vi "test_libssh2_sftp_unlink_ex.vi"() -> ()   [LabVIEW 2017, in "integration_tests.lvlib"]
uses:
  integration_tests.lvlib
  support/support.lvlib
  libssh2/libssh2.lvlib
  <vilib>/PNR/Transparent Assertions/Transparent Assertions/Transparent Assertions.lvlib
panel:
  out "error out":errorcluster
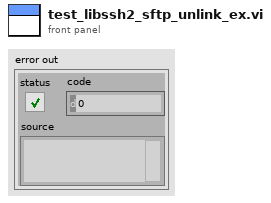
[diagram p1: front panel]
types:
  T1 = typedef "libssh2.lvlib/Session Refnum.ctl" = refnum<k1>
  T2 = typedef "libssh2.lvlib/SFTP Refnum.ctl" = refnum<k1>
  T3 = typedef "libssh2.lvlib/SFTP Handle Refnum.ctl" = refnum<k1>
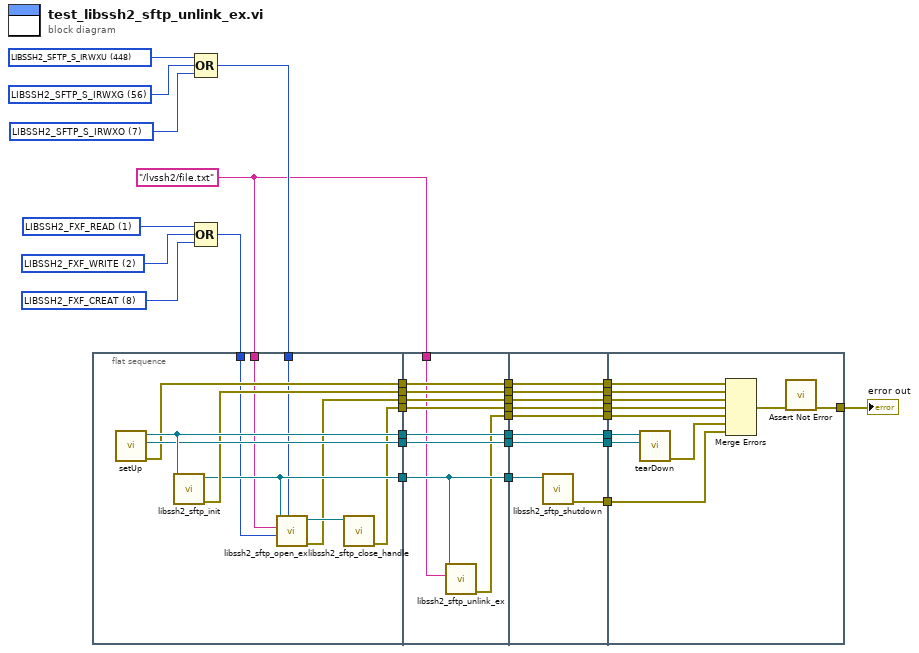
[diagram p0: block diagram]
diagram:
  w27 = u32 2 items=["LIBSSH2_FXF_READ"=1, "LIBSSH2_FXF_WRITE"=2, "LIBSSH2_FXF_APPEND"=4, "LIBSSH2_FXF_CREAT"=8, "LIBSSH2_FXF_TRUNC"=16, "LIBSSH2_FXF_EXCL"=32] ("flags")
  w28 = u32 1 items=["LIBSSH2_FXF_READ"=1, "LIBSSH2_FXF_WRITE"=2, "LIBSSH2_FXF_APPEND"=4, "LIBSSH2_FXF_CREAT"=8, "LIBSSH2_FXF_TRUNC"=16, "LIBSSH2_FXF_EXCL"=32] ("flags")
  w26 = u32 8 items=["LIBSSH2_FXF_READ"=1, "LIBSSH2_FXF_WRITE"=2, "LIBSSH2_FXF_APPEND"=4, "LIBSSH2_FXF_CREAT"=8, "LIBSSH2_FXF_TRUNC"=16, "LIBSSH2_FXF_EXCL"=32] ("flags")
  w3 = "/lvssh2/file.txt" ("filename")
  w30 = 7 items=["LIBSSH2_SFTP_S_IRWXU"=448, "LIBSSH2_SFTP_S_IRUSR"=256, "LIBSSH2_SFTP_S_IWUSR"=128, "LIBSSH2_SFTP_S_IXUSR"=64, "LIBSSH2_SFTP_S_IRWXG"=56, "LIBSSH2_SFTP_S_IRGRP"=32, "LIBSSH2_SFTP_S_IWGRP"=16, "LIBSSH2_SFTP_S_IXGRP"=8, "LIBSSH2_SFTP_S_IRWXO"=7, "LIBSSH2_SFTP_S_IROTH"=4, "LIBSSH2_SFTP_S_IWOTH"=2, "LIBSSH2_SFTP_S_IXOTH"=1] ("mode")
  w31 = 56 items=["LIBSSH2_SFTP_S_IRWXU"=448, "LIBSSH2_SFTP_S_IRUSR"=256, "LIBSSH2_SFTP_S_IWUSR"=128, "LIBSSH2_SFTP_S_IXUSR"=64, "LIBSSH2_SFTP_S_IRWXG"=56, "LIBSSH2_SFTP_S_IRGRP"=32, "LIBSSH2_SFTP_S_IWGRP"=16, "LIBSSH2_SFTP_S_IXGRP"=8, "LIBSSH2_SFTP_S_IRWXO"=7, "LIBSSH2_SFTP_S_IROTH"=4, "LIBSSH2_SFTP_S_IWOTH"=2, "LIBSSH2_SFTP_S_IXOTH"=1] ("mode")
  w32 = 448 items=["LIBSSH2_SFTP_S_IRWXU"=448, "LIBSSH2_SFTP_S_IRUSR"=256, "LIBSSH2_SFTP_S_IWUSR"=128, "LIBSSH2_SFTP_S_IXUSR"=64, "LIBSSH2_SFTP_S_IRWXG"=56, "LIBSSH2_SFTP_S_IRGRP"=32, "LIBSSH2_SFTP_S_IWGRP"=16, "LIBSSH2_SFTP_S_IXGRP"=8, "LIBSSH2_SFTP_S_IRWXO"=7, "LIBSSH2_SFTP_S_IROTH"=4, "LIBSSH2_SFTP_S_IWOTH"=2, "LIBSSH2_SFTP_S_IXOTH"=1] ("mode")
  n1 = flat-sequence {
    tunnel: [w44] -> w14
    tunnel: [w43] -> w13
    tunnel: [w40] -> w12
    tunnel: [w42] -> w11
    tunnel: [w41] -> w10
    tunnel: w29 -> [w39]
    tunnel: w3 -> [w38]
    tunnel: w25 -> [w37]
    tunnel: [w35] -> w9
    tunnel: [w34] -> w4
    tunnel: [w53] -> w19
    tunnel: [w52] -> w18
    tunnel: [w51] -> w17
    tunnel: [w50] -> w16
    tunnel: [w49] -> w15
    tunnel: [w48] -> w8
    tunnel: [w47] -> w5
    tunnel: w3 -> [w46]
    tunnel: w4 -> [w47]
    tunnel: w9 -> [w48]
    tunnel: w10 -> [w49]
    tunnel: w11 -> [w50]
    tunnel: w12 -> [w51]
    tunnel: w13 -> [w52]
    tunnel: w14 -> [w53]
    tunnel: [w45] -> w2
    tunnel: w19 -> [w62]
    tunnel: [w62] -> w24
    tunnel: w18 -> [w61]
    tunnel: [w61] -> w23
    tunnel: w17 -> [w58]
    tunnel: w16 -> [w60]
    tunnel: [w60] -> w22
    tunnel: w15 -> [w59]
    tunnel: [w59] -> w21
    tunnel: [w57] -> w20
    tunnel: w8 -> [w56]
    tunnel: [w56] -> w7
    tunnel: [w55] -> w6
    tunnel: w5 -> [w55]
    tunnel: w2 -> [w54]
    tunnel: [w54] -> w1
    tunnel: w24 -> [w73]
    tunnel: w23 -> [w72]
    tunnel: w22 -> [w71]
    tunnel: [w68] -> w33
    tunnel: w21 -> [w67]
    tunnel: w20 -> [w66]
    tunnel: w7 -> [w65]
    tunnel: w6 -> [w64]
    tunnel: w1 -> [w63]
    frame #0 {
      n2 = call "setUp.vi"() -> ("error out"=w42:errorcluster, "connection ID"=w43:refnum<k5>, "session"=w44:T1)  [unwired: 9 in]
      n3 = call "libssh2_sftp_init.vi"("session"=w44) -> ("error out"=w41:errorcluster, "sftp"=w40:T2)  [unwired: 9 in]
      n4 = call "libssh2_sftp_open_ex.vi"("mode"=w39, "flags"=w37, "filename"=w38, "sftp"=w40) -> ("error out"=w35:errorcluster, "sftp handle"=w36:T3)  [unwired: 6 in]
      n5 = call "libssh2_sftp_close_handle.vi"("sftp handle"=w36) -> ("error out"=w34:errorcluster)  [unwired: 10 in]
    }
    frame #1 {
      n6 = call "libssh2_sftp_unlink_ex.vi"("file"=w46, "sftp"=w51) -> ("error out"=w45:errorcluster)  [unwired: 9 in]
    }
    frame #2 {
      n7 = call "libssh2_sftp_shutdown.vi"("sftp"=w58) -> ("error out"=w57:errorcluster)  [unwired: 10 in]
    }
    frame #3 {
      n8 = call "tearDown.vi"("connection ID"=w72, "session"=w73) -> ("error out"=w70:errorcluster)  [unwired: 9 in]
      n9 = Merge Errors(w71, w67, w65, w64, w63, w70, w66) -> (w69:errorcluster)
      n10 = call <vilib>:"Assert Not Error.vi"("error in (no error)"=w69) -> ("error out"=w68:errorcluster)  [unwired: 10 in]
    }
  }
  n11 = Compound Arithmetic op=OR(w32, w31, w30) -> (w29:i32)
  n12 = Compound Arithmetic op=OR(w28, w27, w26) -> (w25:u32)
  "error out" <- w33
